vi "Bundle.vi"() -> ()   [LabVIEW 2016]
panel:
  out "appended array":dbl[](array[numeric])
  out "output cluster":T1
  in  "String":string
  in  "Boolean":bool
  in  "Numeric Control 2":dbl
  in  "Numeric Control":dbl
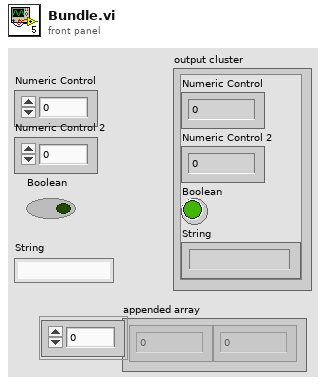
[diagram p1: front panel]
types:
  T1 = cluster{"Numeric Control":dbl, "Numeric Control 2":dbl, "Boolean":bool, "String":string}
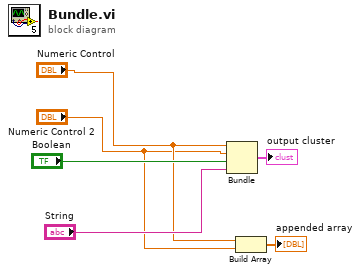
[diagram p0: block diagram]
diagram:
  n1 = Bundle("Numeric Control"="Numeric Control", "Numeric Control 2"="Numeric Control 2", "Boolean"="Boolean", "String"="String") -> (→"output cluster":T1)  [unwired: 1 in]
  n2 = Build Array("Numeric Control", "Numeric Control 2") -> (→"appended array":dbl[])
